vi "Replace_Subtrack_for_Special_Case-1-1.vi"(4 "error IN":errorcluster, 5 "[IN] Special case?":bool, 7 "[IN] Subtracks":T1(array[cluster])) -> (0 "error OUT":errorcluster, 1 "[OUT Special case?":bool, 3 "[OUT] Subtracks":T1(array[cluster]))   [LabVIEW 2013]
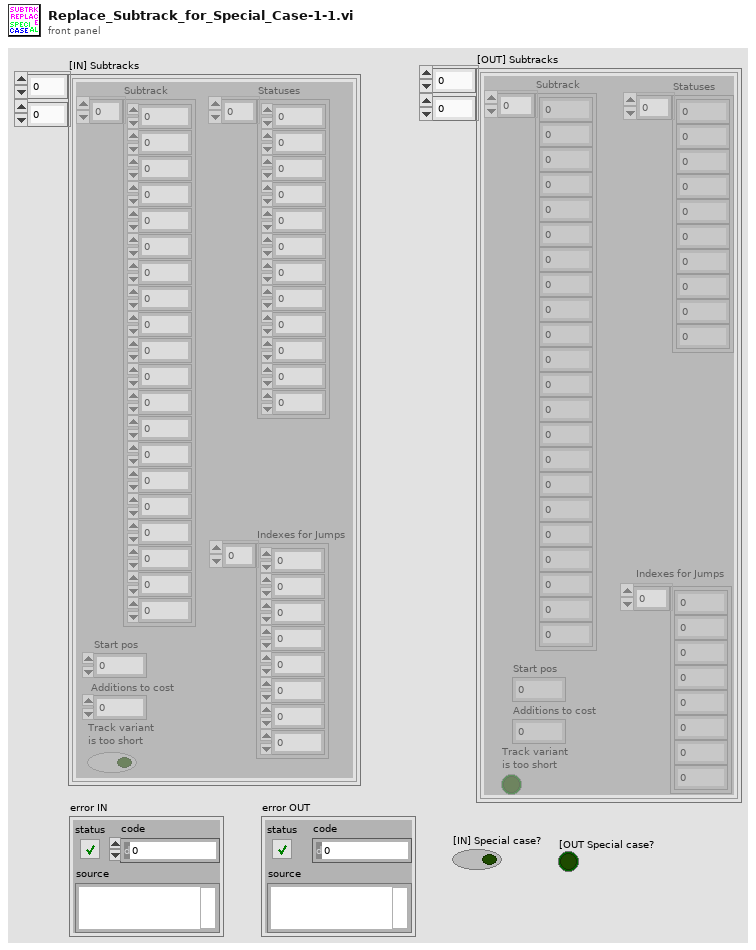
[diagram p1: front panel]
types:
  T1 = cluster{"Subtrack":dbl[], "Statuses":i16[], "Start pos":i32, "Additions to cost":i32, "Track variant \nis too short":bool, "Indexes for Jumps":i32[]}[][]
  T2 = cluster{"Subtrack":dbl[], "Statuses":i16[], "Start pos":i32, "Additions to cost":i32, "Track variant \nis too short":bool, "Indexes for Jumps":i32[]}[]
  T3 = cluster{"Subtrack":dbl[], "Statuses":i16[], "Start pos":i32, "Additions to cost":i32, "Track variant \nis too short":bool, "Indexes for Jumps":i32[]}
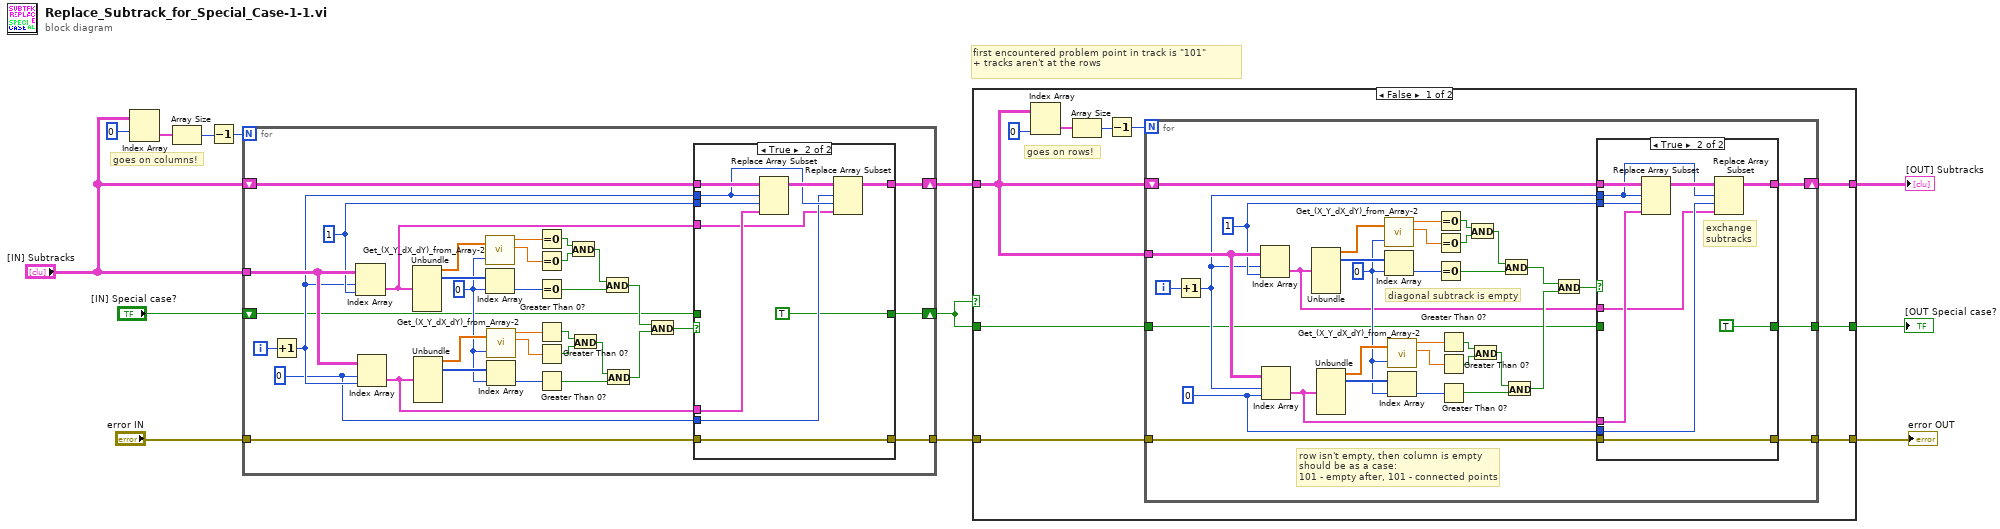
[diagram p0: block diagram]
diagram:
  # "goes on columns!"
  # "first encountered problem point in track is \"101\"\n+ tracks aren't at the rows"
  n1 = Index Array(array="[IN] Subtracks", index (row)=0 ("disabled index (col)")) -> (element=w9:T2)  [unwired: 1 in]
  n2 = Array Size(array=w9) -> (size(s)=w8:i32)
  n3 = Decrement(x=w8) -> (x-1=w7:i32)
  n4 = for {
    N: w7 -> [_]
    tunnel: "[IN] Subtracks" -> [w47]
    shift-right: [w18] -> w12
    shift-left: "[IN] Subtracks" -> [w24]
    tunnel: "error IN" -> [w17]
    tunnel: [w16] -> w11
    shift-right: [w14] -> w13
    shift-left: "[IN] Special case?" -> [w15]
    i -> [w48]
    w32 = 0 ("index")
    w19 = 0 ("disabled index (col)")
    w21 = 1 ("disabled index (col)")
    n5 = Increment(x=w48) -> (x+1=w20:i32)
    n6 = Index Array(array=w47, index (row)=w20, index (col)=w21) -> (element=w23:T3)
    n7 = Index Array(array=w47, index (row)=w19, index (col)=w20) -> (element=w22:T3)
    n8 = Unbundle(w23) -> ("Subtrack"=w44:dbl[], "Statuses"=w46:i16[])  [unwired: 4 out]
    n9 = Unbundle(w22) -> ("Subtrack"=w43:dbl[], "Statuses"=w45:i16[])  [unwired: 4 out]
    n10 = call "Get_(X_Y_dX_dY)_from_Array-2.vi"("(X,Y,dX,dY)"=w44, "Index of Displacement"=w32) -> ("X"=w42:dbl, "Y"=w41:dbl)  [unwired: 2 out]
    n11 = Index Array(array=w46, index=w32) -> (element=w40:i16)
    n12 = call "Get_(X_Y_dX_dY)_from_Array-2.vi"("(X,Y,dX,dY)"=w43, "Index of Displacement"=w32) -> ("X"=w35:dbl, "Y"=w34:dbl)  [unwired: 2 out]
    n13 = Index Array(array=w45, index=w32) -> (element=w33:i16)
    n14 = Equal To 0?(x=w42) -> (x = 0?=w39:bool)
    n15 = Equal To 0?(x=w41) -> (x = 0?=w38:bool)
    n16 = Equal To 0?(x=w40) -> (x = 0?=w36:bool)
    n17 = Greater Than 0?(x=w35) -> (x > 0?=w31:bool)
    n18 = Greater Than 0?(x=w34) -> (x > 0?=w30:bool)
    n19 = Greater Than 0?(x=w33) -> (x > 0?=w28:bool)
    n20 = And(x=w39, y=w38) -> (x .and. y?=w37:bool)
    n21 = And(x=w31, y=w30) -> (x .and. y?=w29:bool)
    n22 = And(x=w37, y=w36) -> (x .and. y?=w27:bool)
    n23 = And(x=w29, y=w28) -> (x .and. y?=w26:bool)
    n24 = And(x=w27, y=w26) -> (x .and. y?=w25:bool)
    n25 = case shown="True" w25 {
      tunnel: w24 -> [w51 w61]
      tunnel: w23 -> [_ w55]
      tunnel: w22 -> [_ w59]
      tunnel: w20 -> [_ w57]
      tunnel: w21 -> [_ w60]
      tunnel: w19 -> [_ w56]
      tunnel: [w51 w54] -> w18
      tunnel: w17 -> [w50 w53]
      tunnel: [w50 w53] -> w16
      tunnel: w15 -> [w49 _]
      tunnel: [w49 TRUE] -> w14
      frame False {
      }
      frame True {
        n26 = Replace Array Subset(array=w61, new element=w59, index (row)=w57, index (col)=w60) -> (w58:T1)
        n27 = Replace Array Subset(array=w58, new element=w55, index (row)=w56, index (col)=w57) -> (w54:T1)
      }
    }
  }
  n28 = case shown="False" w13 {
    tunnel: w12 -> [w67 w122]
    tunnel: w11 -> [w65 w120]
    tunnel: w13 -> [w66 w121]
    tunnel: [w64 w122] -> w1
    tunnel: [w63 w121] -> w10
    tunnel: [w62 w120] -> w2
    frame False {
      # "goes on rows!"
      n29 = Index Array(array=w67, index (col)=0 ("index (row)")) -> (element=w70:T2)  [unwired: 1 in]
      n30 = Array Size(array=w70) -> (size(s)=w71:i32)
      n31 = Decrement(x=w71) -> (x-1=w69:i32)
      n32 = for {
        N: w69 -> [_]
        shift-right: [w75] -> w64
        shift-left: w67 -> [w82]
        tunnel: w67 -> [w96]
        tunnel: w66 -> [w74]
        tunnel: w65 -> [w80]
        tunnel: [w73] -> w63
        tunnel: [w72] -> w62
        i -> [w106]
        w77 = 0 ("disabled index (col)")
        w86 = 0 ("index")
        w79 = 1 ("disabled index (col)")
        # "row isn't empty, then column is empty\nshould be as a case:\n101 - empty after, 101 - connected points"
        # "diagonal subtrack is empty"
        n33 = Increment(x=w106) -> (x+1=w78:i32)
        n34 = Index Array(array=w96, index (row)=w78, index (col)=w79) -> (element=w76:T3)
        n35 = Index Array(array=w96, index (row)=w78, index (col)=w77) -> (element=w81:T3)
        n36 = Unbundle(w76) -> ("Subtrack"=w104:dbl[], "Statuses"=w105:i16[])  [unwired: 4 out]
        n37 = Unbundle(w81) -> ("Subtrack"=w94:dbl[], "Statuses"=w95:i16[])  [unwired: 4 out]
        n38 = call "Get_(X_Y_dX_dY)_from_Array-2.vi"("(X,Y,dX,dY)"=w104, "Index of Displacement"=w86) -> ("X"=w103:dbl, "Y"=w102:dbl)  [unwired: 2 out]
        n39 = Index Array(array=w105, index=w86) -> (element=w101:i16)
        n40 = call "Get_(X_Y_dX_dY)_from_Array-2.vi"("(X,Y,dX,dY)"=w94, "Index of Displacement"=w86) -> ("X"=w93:dbl, "Y"=w92:dbl)  [unwired: 2 out]
        n41 = Index Array(array=w95, index=w86) -> (element=w91:i16)
        n42 = Equal To 0?(x=w103) -> (x = 0?=w100:bool)
        n43 = Equal To 0?(x=w102) -> (x = 0?=w99:bool)
        n44 = Equal To 0?(x=w101) -> (x = 0?=w97:bool)
        n45 = Greater Than 0?(x=w93) -> (x > 0?=w90:bool)
        n46 = Greater Than 0?(x=w92) -> (x > 0?=w89:bool)
        n47 = Greater Than 0?(x=w91) -> (x > 0?=w87:bool)
        n48 = And(x=w100, y=w99) -> (x .and. y?=w98:bool)
        n49 = And(x=w90, y=w89) -> (x .and. y?=w88:bool)
        n50 = And(x=w98, y=w97) -> (x .and. y?=w85:bool)
        n51 = And(x=w88, y=w87) -> (x .and. y?=w84:bool)
        n52 = And(x=w85, y=w84) -> (x .and. y?=w83:bool)
        n53 = case shown="True" w83 {
          tunnel: w82 -> [w108 w119]
          tunnel: w81 -> [_ w117]
          tunnel: w80 -> [w109 w111]
          tunnel: w79 -> [_ w118]
          tunnel: w78 -> [_ w114]
          tunnel: w77 -> [_ w115]
          tunnel: w76 -> [_ w113]
          tunnel: [w108 w112] -> w75
          tunnel: [w109 w111] -> w72
          tunnel: w74 -> [w107 _]
          tunnel: [w107 TRUE] -> w73
          frame False {
          }
          frame True {
            # "exchange \nsubtracks"
            n54 = Replace Array Subset(array=w119, new element=w117, index (row)=w114, index (col)=w118) -> (w116:T1)
            n55 = Replace Array Subset(array=w116, new element=w113, index (row)=w114, index (col)=w115) -> (w112:T1)
          }
        }
      }
    }
    frame True {
    }
  }
  "error OUT" <- w2
  "[OUT] Subtracks" <- w1
  "[OUT Special case?" <- w10
